vi "Write all steps to sequence file.vi"(0 "User input 1":T1, 5 "Sequence":T2[](array[typedef]), 7 "Sequence name":string, 11 "error in (no error)":errorcluster) -> (15 "error out":errorcluster)   [LabVIEW 2011]
uses:
  Sequence steps config..ctl
  Single criteria cluster.ctl
  Criteria types.ctl
  Boolean operation.ctl
  User input.ctl
  <vilib>/Utility/libraryn.llb/Check if File or Folder Exists.vi
  <vilib>/Utility/config.llb/NI_LVConfig.lvlib
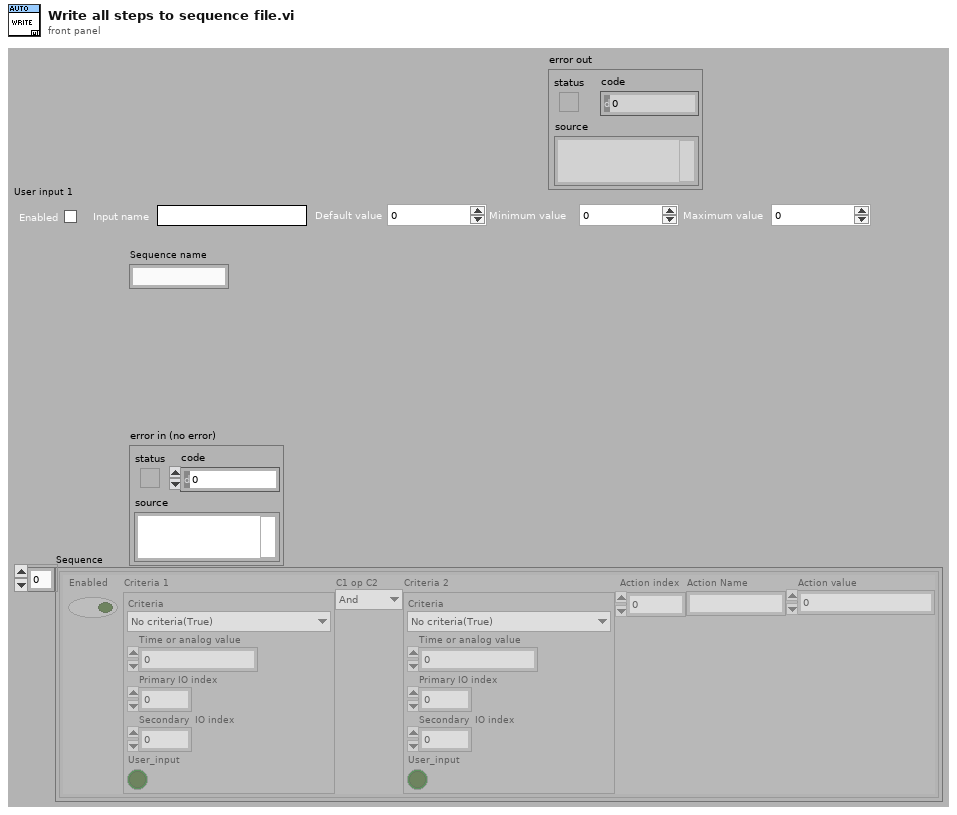
[diagram p1: front panel]
types:
  T1 = typedef "User input.ctl" = cluster{"Input name":string, "Minimum value ":dbl, "Maximum value":dbl, "Default value":dbl, "User inp enabled":bool}
  T2 = typedef "Sequence steps config..ctl" = cluster{"Enabled":bool, "Criteria 1":T3, "C1 op C2":T5, "Criteria 2":T3, "Action index":i32, "Action Name":string, "Action value":dbl}
  T3 = typedef "Single criteria cluster.ctl" = cluster{"Criteria":T4, "Time or analog value":dbl, "Primary IO index":i32, "Secondary  IO index":i32, "User_input":bool}
  T4 = typedef "Criteria types.ctl" = enum16{"No criteria(True)", "Time(s)", "Analog IO over", "Analog IO over or equal", "Analog IO under", "Analog IO under or equal", "Analog IO 1 minus Analog IO 2 over", "Digital IO True", "Digital IO False", "Operator approval"}
  T5 = typedef "Boolean operation.ctl" = enum16{"And", "Or", "Xor", "Nand", "Nor", "Nxor", "Implies"}
  T6 = typedef "NI_LVConfig.lvlib/Config Data RefNum.ctl" = refnum<k1>
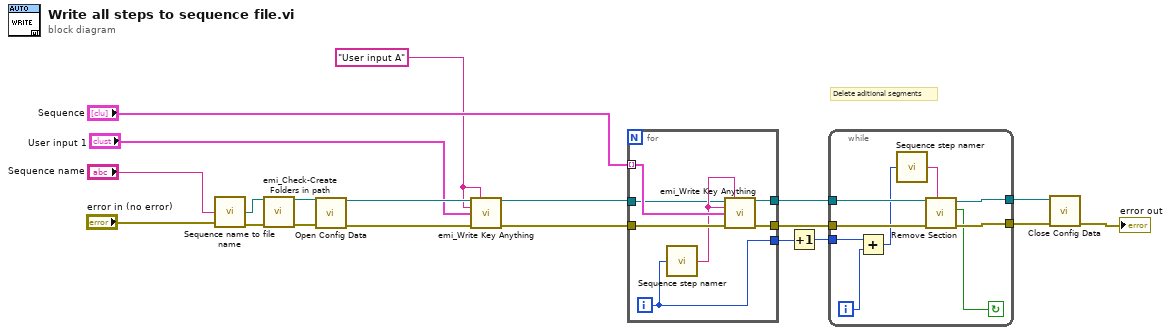
[diagram p0: block diagram]
diagram:
  w2 = "User input A" ("Section(Default)")
  # "Delete aditional segments"
  n1 = call "Sequence name to file name.vi"("Sequence name"="Sequence name", "error in (no error)"="error in (no error)") -> ("Sequence file path"=w18:path, "error out"=w17:errorcluster)  [unwired: 12 in]
  n2 = call "emi_Check-Create Folders in path.vi"("Path including file"=w18, "error in (no error)"=w17) -> ("Path out"=w15:path, "error out"=w16:errorcluster)  [unwired: 11 in, 1 out]
  n3 = call <vilib>:"Open Config Data.vi"("error in (no error)"=w16, "configuration file path"=w15) -> ("error out"=w6:errorcluster, "refnum"=w4:T6)  [unwired: 7 in, 1 out]
  n4 = call "emi_Write Key Anything.vi"("Ini file refnum"=w4, "Section(Default)"=w2, "Name"=w2, "Anything"="User input 1", "error in (no error)"=w6) -> ("Ini file refnum out"=w3:T6, "error out"=w5:errorcluster)  [unwired: 9 in]
  n5 = for {
    tunnel: w5 -> [w27]
    tunnel: "Sequence" -> [w26] mode=indexing
    tunnel: [w24] -> w12
    tunnel: [w23] -> w13
    tunnel: w3 -> [w22]
    tunnel: [w21] -> w10
    i -> [w24]
    n6 = call "Sequence step namer.vi"("number"=w24) -> ("Step name"=w25:string)
    n7 = call "emi_Write Key Anything.vi"("Ini file refnum"=w22, "Section(Default)"=w25, "Name"=w25, "Anything"=w26, "error in (no error)"=w27) -> ("Ini file refnum out"=w21:T6, "error out"=w23:errorcluster)  [unwired: 9 in]
  }
  n8 = Increment(x=w12) -> (x+1=w11:i32)
  n9 = while {
    tunnel: w13 -> [w36]
    tunnel: w11 -> [w35]
    tunnel: w10 -> [w33]
    tunnel: [w30] -> w9
    tunnel: [w29] -> w8
    i -> [w34]
    stop <- w28 continue-if-true
    n10 = Add(x=w35, y=w34) -> (x+y=w32:i32)
    n11 = call "Sequence step namer.vi"("number"=w32) -> ("Step name"=w31:string)
    n12 = call <vilib>:"Remove Section.vi"("section"=w31, "error in (no error)"=w36, "refnum"=w33) -> ("error out"=w30:errorcluster, "section exists?"=w28:bool, "refnum out"=w29:T6)  [unwired: 6 in]
  }
  n13 = call <vilib>:"Close Config Data.vi"("error in (no error)"=w9, "refnum"=w8) -> ("error out"=→"error out":errorcluster)  [unwired: 8 in, 1 out]
